vi "DI-handler.vi"(9 "hex integer string in":string, 11 "Current DI State":T1) -> (1 "input state changed":bool, 3 "New DI State":T1)   [LabVIEW 2024]
uses:
  controls/digitial-input-cluster.ctl
panel:
  out "re-combobulated number":u32
  out "hex integer string":string
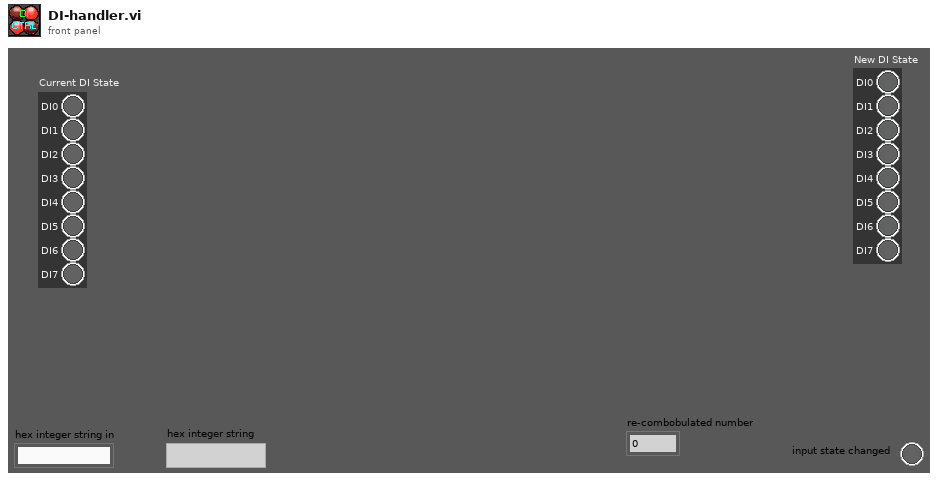
[diagram p1: front panel]
types:
  T1 = typedef "digitial-input-cluster.ctl" = cluster{"DI0":bool, "DI1":bool, "DI2":bool, "DI3":bool, "DI4":bool, "DI5":bool, "DI6":bool, "DI7":bool}
  T2 = cluster{"Boolean array[0]":bool, "Boolean array[1]":bool, "Boolean array[2]":bool, "Boolean array[3]":bool, "Boolean array[4]":bool, "Boolean array[5]":bool, "Boolean array[6]":bool, "Boolean array[7]":bool, "Boolean array[8]":bool}
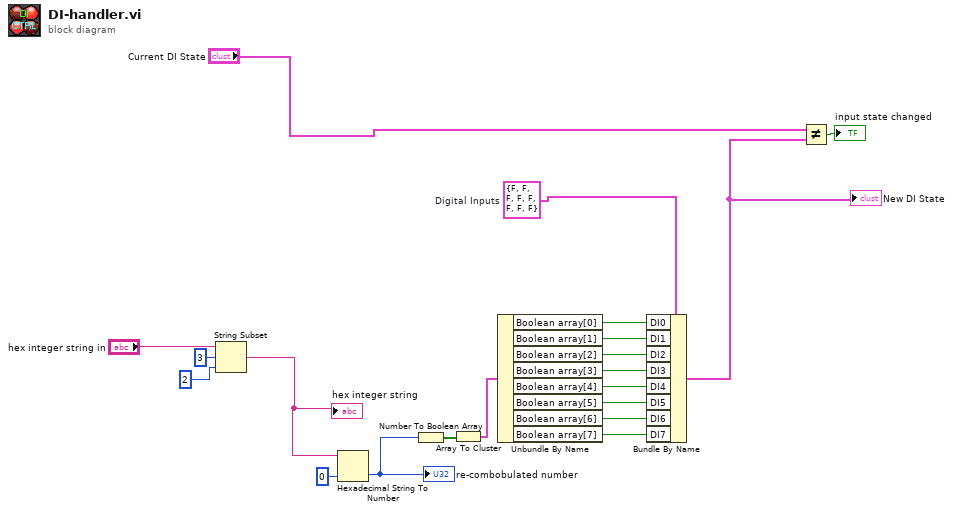
[diagram p0: block diagram]
diagram:
  w1 = T1 {"DI0"=FALSE, "DI1"=FALSE, "DI2"=FALSE, "DI3"=FALSE, "DI4"=FALSE, "DI5"=FALSE, "DI6"=FALSE, "DI7"=FALSE}  # Digital Inputs
  n1 = String Subset(string="hex integer string in", offset (0)=3, length (rest)=2 ("length (rest)")) -> (substring=w4:string)
  "hex integer string" <- w4
  n2 = Hexadecimal String To Number(string=w4, default (0uL)=u32 0 ("default (0 U32)")) -> (number=w18:u32)  [unwired: 1 in, 1 out]
  "re-combobulated number" <- w18
  n3 = Number To Boolean Array(number=w18) -> (Boolean array=w17:bool[])
  n4 = Array To Cluster(array=w17) -> (cluster=w16:T2)
  n5 = Unbundle By Name(w16) -> ("Boolean array[0]"=w15:bool, "Boolean array[1]"=w14:bool, "Boolean array[2]"=w13:bool, "Boolean array[3]"=w12:bool, "Boolean array[4]"=w11:bool, "Boolean array[5]"=w10:bool, "Boolean array[6]"=w9:bool, "Boolean array[7]"=w8:bool)
  n6 = Bundle By Name(cluster=w1, "DI0"=w15, "DI1"=w14, "DI2"=w13, "DI3"=w12, "DI4"=w11, "DI5"=w10, "DI6"=w9, "DI7"=w8) -> (w2:T1)
  "New DI State" <- w2
  n7 = Not Equal?(x="Current DI State", y=w2) -> (x != y?=→"input state changed":bool)
